vi "Current-Timestamp (SubVI).vi"(11 "Extension":string) -> (3 "Path":path)   [LabVIEW 2020]
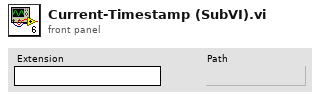
[diagram p1: front panel]
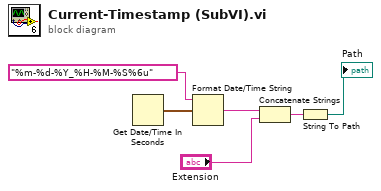
[diagram p0: block diagram]
diagram:
  n1 = Get Date/Time In Seconds() -> (seconds since 1Jan1904=w1:timestamp)
  n2 = Format Date/Time String(time format string (%c)="%m-%d-%Y_%H-%M-%S%6u", seconds (now)=w1) -> (date/time string=w3:string)  [unwired: 1 in]
  n3 = Concatenate Strings(w3, "Extension") -> (w4:string)
  n4 = String To Path(string=w4) -> (path=→"Path":path)
